vi "Unit Test.vi"() -> ()   [LabVIEW 2019, in "Fluidic Process.lvlib"]
uses:
  Fluidic Process.lvlib
  SubVI/Fluidic Para.ctl
  User Event/Controls/UE Abort Action.ctl
  <vilib>/Utility/file.llb/Read Delimited Spreadsheet (string).vi
  Syringe Pump/NE-500/NE-500.lvlib
  Selection Valve/IDEX/IDEX.lvlib
  LED/LED.lvlib
  IO/sbRIO9623/sbRIO9623.lvlib
panel:
  out "Force Sensor":bool
  out "Air Sealing":bool
  out "Total Process":string
  out "Current Process":string
  out "Remaining Time(s)":dbl
  out "Gauge":dbl(knob)=1.2869315802184793e-48 scale=0.0..101.0
  in  "File Path":path
  in  "Fluidic Para":T1
  in  "Stop":bool
  in  "Run":bool
  out "Syringe Pump":bool
  out "Selection Valve":bool
  out "LED":bool
  out "I/O":bool
  in  "Open":bool
  # "/"
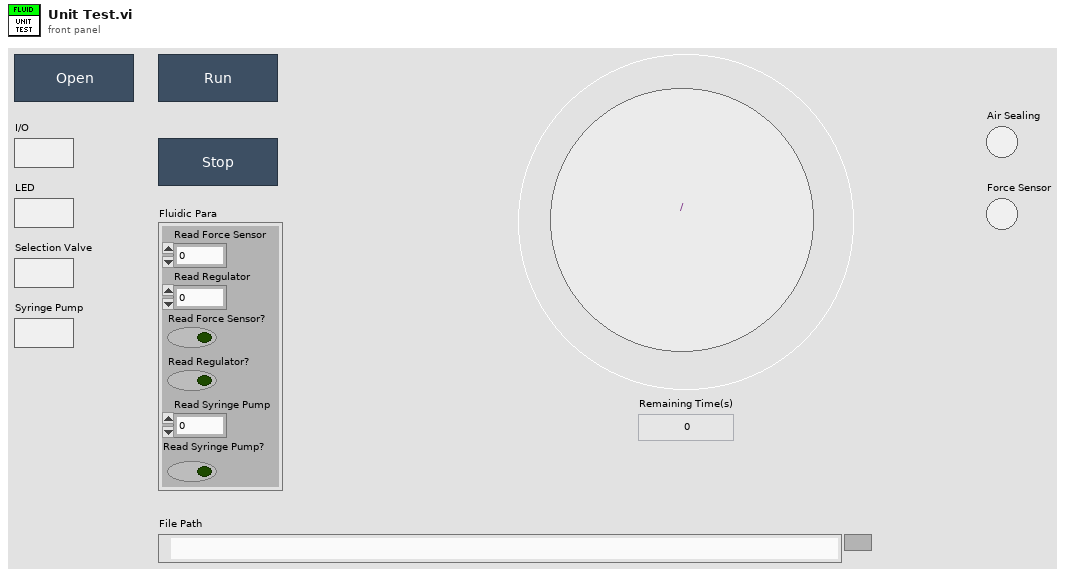
[diagram p1: front panel]
types:
  T1 = typedef "Fluidic Process.lvlib/Fluidic Para.ctl" = cluster{"Read Force Sensor":i32, "Read Regulator":i32, "Read Force Sensor?":bool, "Read Regulator?":bool, "Read Syringe Pump":i32, "Read Syringe Pump?":bool}
  T2 = typedef "UE Abort Action.ctl" = enum16{"Create", "Get", "Destroy"}
  T3 = typedef "Fluidic Process.lvlib/SEQ Data.ctl" = cluster{"Fluidic Process Done?":bool, "Current Process":i32, "Remaining Time":dbl, "Total Process":i32, "Air Sealing":bool, "Force Condition":bool}
  T4 = typedef "sbRIO9623.lvlib/SEQ Data.ctl" = cluster{"Lid Sensor 1":bool, "Lid Sensor 2":bool, "Laser Interlock":bool, "Buffer Tank":bool, "Wash Tank":bool, "Waste Tank":bool, "SiPM 1":fxp<+,20,5>, "SiPM 2":fxp<+,20,5>, "Initialize Success?":bool, "VI Refnum":refnum<vi>}
  T5 = typedef "LED.lvlib/SEQ Data.ctl" = cluster{"Initialize Sucess?":bool, "BL2 Regulator":dbl, "BL1 Regulator":dbl, "Blood Sensor 1":dbl, "Blood Sensor 2":dbl, "Air Pressure Sensor":dbl, "Force Snesor 1":u32, "Force Snesor 2":u32, "VI Refnum":refnum<vi>}
  T6 = typedef "IDEX.lvlib/SEQ Data.ctl" = cluster{"Position":string, "Initialize Done?":bool, "VI Refnum":refnum<vi>}
  T7 = typedef "NE-500.lvlib/SEQ Data.ctl" = cluster{"Status":string, "Initialize Done?":bool, "VI Refnum":refnum<vi>}
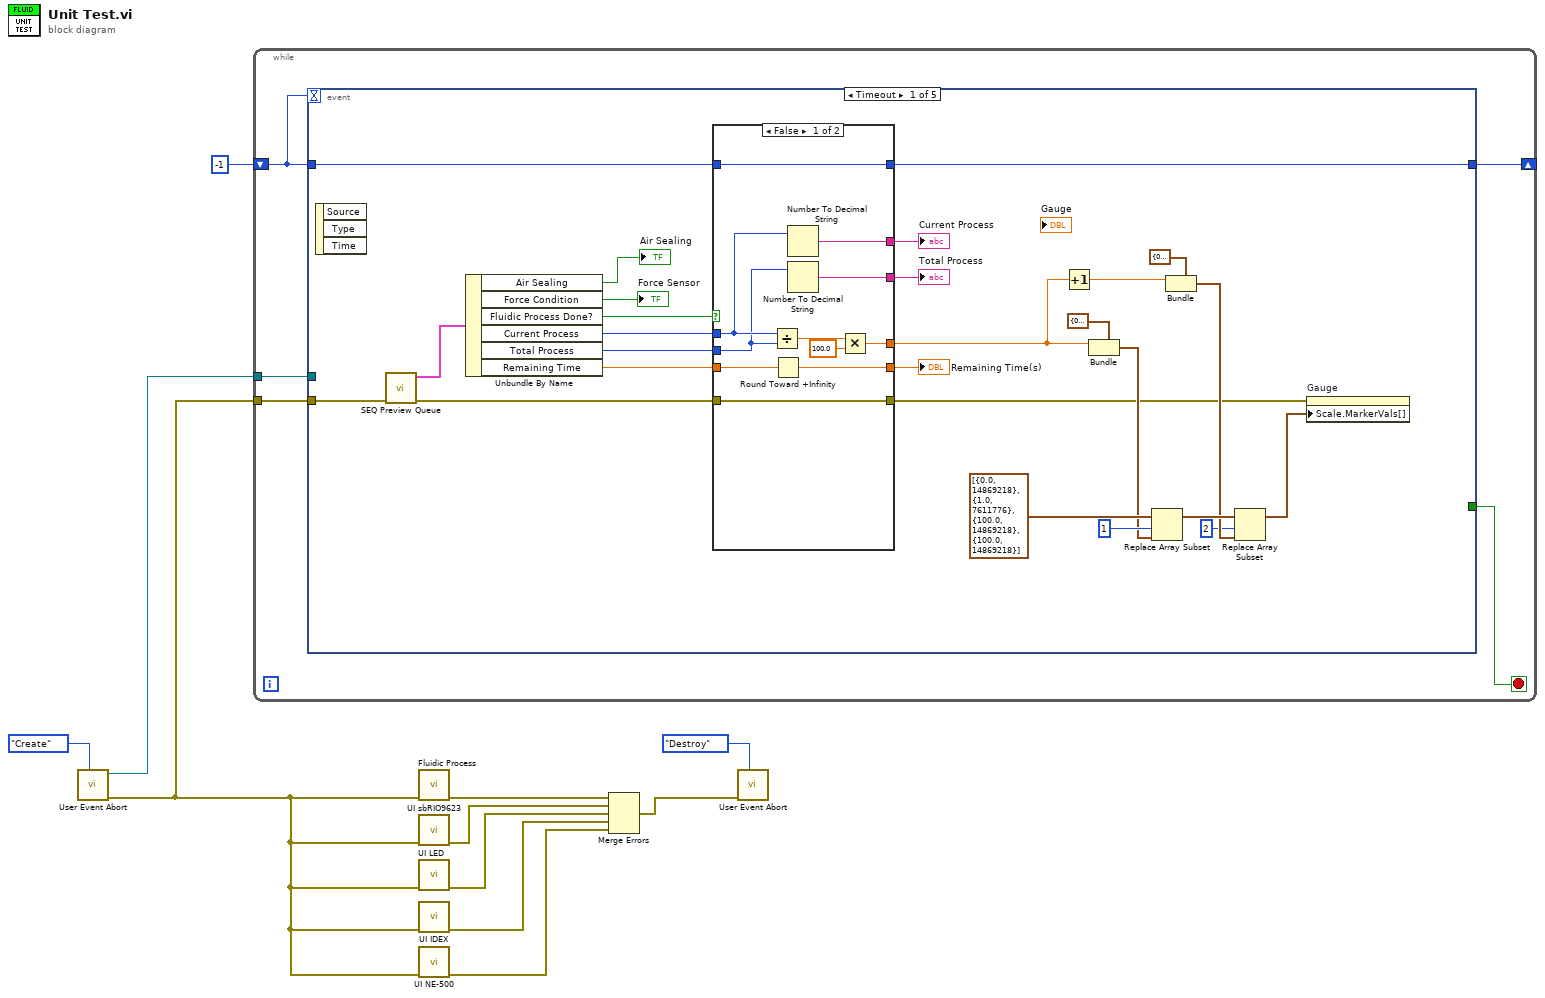
[diagram p0: block diagram]
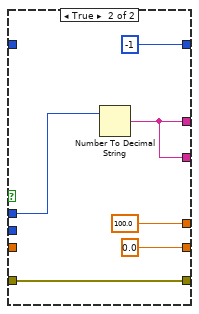
[diagram p2: hidden frame]
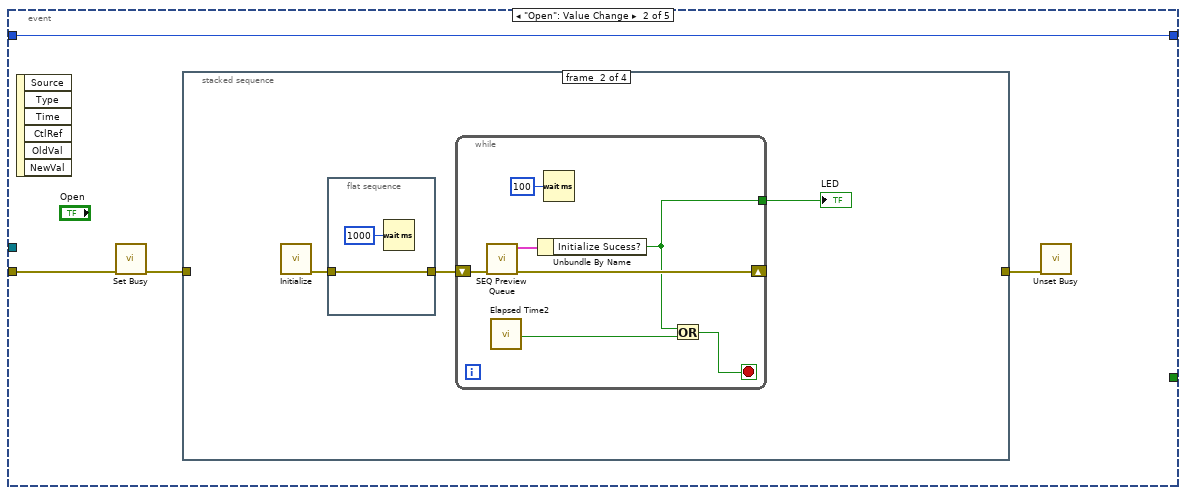
[diagram p3: hidden frame]
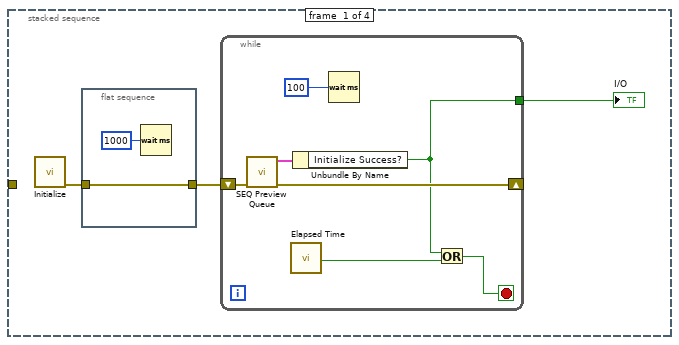
[diagram p4: hidden frame]
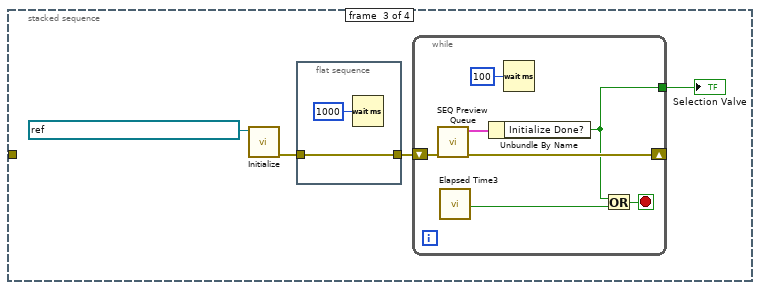
[diagram p5: hidden frame]
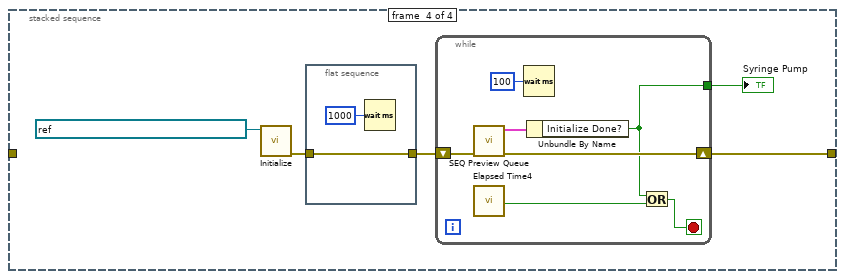
[diagram p6: hidden frame]
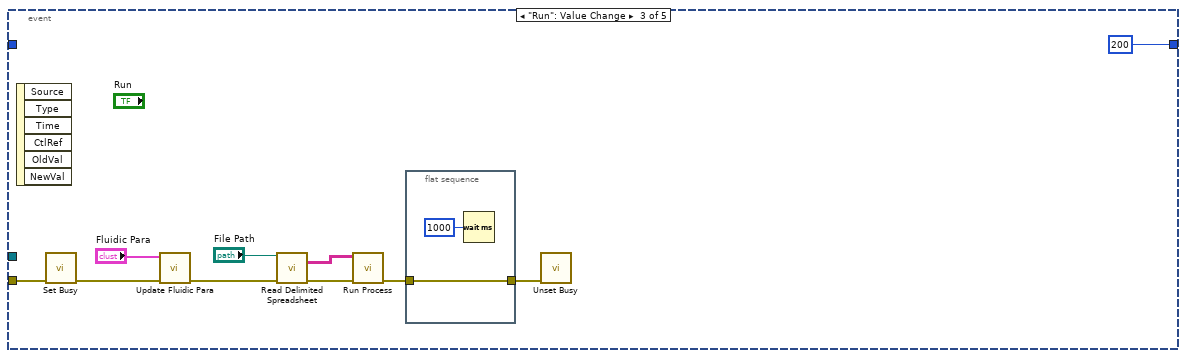
[diagram p7: hidden frame]
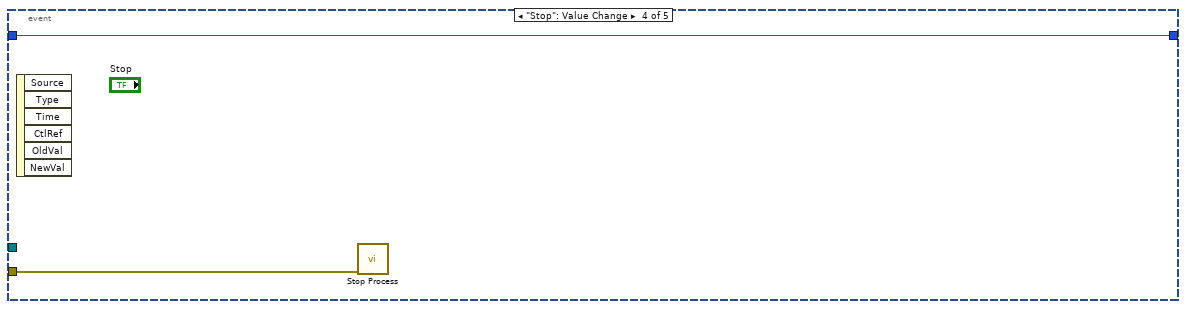
[diagram p8: hidden frame]
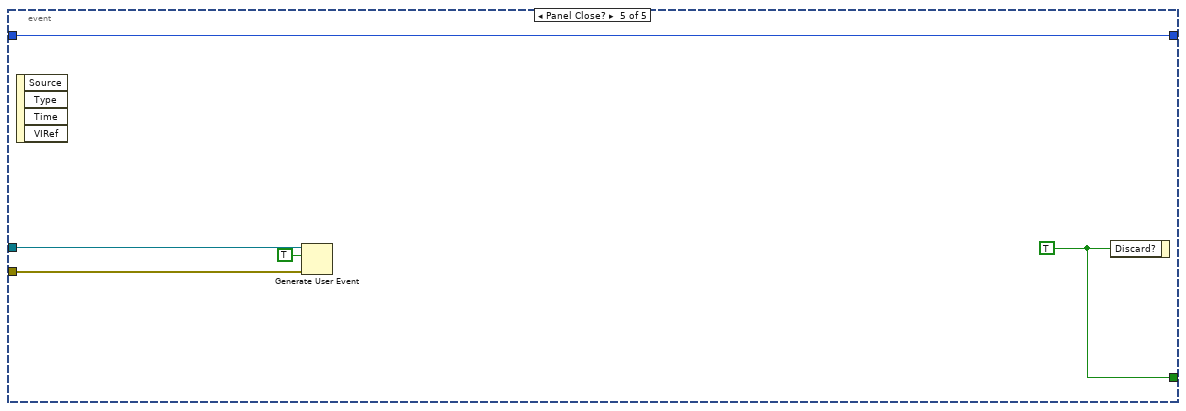
[diagram p9: hidden frame]
diagram:
  n1 = call "User Event Abort.vi"("Action"=UE_Abort_Action."Create") -> ("Error Out"=w2:errorcluster, "User Event Out"=w3:refnum<user-event>)  [unwired: 9 in]
  n2 = while {
    tunnel: w3 -> [w16]
    tunnel: w2 -> [w15]
    shift-right: [w13] -> _
    shift-left: -1 -> [w12]
    stop <- w14 stop-if-true
    n3 = event shown="[0] Timeout" {
      selector: _ -> [_ _ _ _ _]
      dyn-events: _ -> [_ _ _ _ _]
      timeout: w12 -> [_ _ _ _ _]
      tunnel: w16 -> [_ _ _ _ w133]
      tunnel: w15 -> [w42 w63 w118 w127 w132]
      tunnel: [_ _ _ _ w130] -> w14
      tunnel: w12 -> [w35 w60 _ w128 w129]
      tunnel: [w34 w60 200 w128 w129] -> w13
      event Timeout {
        n4 = event-data() -> ()  [unwired: 1 in, 3 out]
        n5 = call "SEQ Preview Queue.vi"("error in"=w42) -> ("error out"=w40:errorcluster, "SEQ Data"=w41:T3)  [unwired: 9 in]
        n6 = Unbundle By Name(w41) -> ("Air Sealing"=→"Air Sealing":bool, "Force Condition"=→"Force Sensor":bool, "Fluidic Process Done?"=w39:bool, "Current Process"=w38:i32, "Total Process"=w37:i32, "Remaining Time"=w36:dbl)
        n7 = case shown="False" w39 {
          tunnel: w40 -> [w49 w56]
          tunnel: w38 -> [w48 w55]
          tunnel: w37 -> [w46 _]
          tunnel: w36 -> [w44 _]
          tunnel: [w43 0.0 ("Remaining Time")] -> w21
          tunnel: [w51 100.0] -> w23
          tunnel: w35 -> [w50 _]
          tunnel: [w50 -1] -> w34
          tunnel: [w49 w56] -> w22
          tunnel: [w47 w54] -> w20
          tunnel: [w45 w54] -> w19
          frame False {
            n8 = Divide(x=w48, y=w46) -> (x/y=w53:dbl)
            n9 = Round Toward +Infinity(x=w44) -> (ceil(x): smallest int >= x=w43:dbl)
            n10 = Number To Decimal String(number=w48) -> (decimal integer string=w47:string)  [unwired: 1 in]
            n11 = Number To Decimal String(number=w46) -> (decimal integer string=w45:string)  [unwired: 1 in]
            n12 = Multiply(x=w53, y=100.0) -> (x*y=w51:dbl)
          }
          frame True {
            n13 = Number To Decimal String(number=w55) -> (decimal integer string=w54:string)  [unwired: 1 in]
          }
        }
        "Remaining Time(s)" <- w21
        "Current Process" <- w20
        "Total Process" <- w19
        n14 = Increment(x=w23) -> (x+1=w29:dbl)
        n15 = Bundle(cluster=cluster{dbl, i32} {0.0, 7611776}, w23) -> (w31:cluster{dbl, i32})  [unwired: 1 in]
        n16 = Replace Array Subset(array=cluster{dbl, u32}[] [{0.0, 14869218}, {1.0, 7611776}, {100.0, 14869218}, {100.0, 14869218}] ("Scale.Marker Values[]"), new element=w31, index=1) -> (w27:cluster{dbl, u32}[])
        n17 = Bundle(cluster=cluster{dbl, i32} {0.0, 14869218}, w29) -> (w26:cluster{dbl, i32})  [unwired: 1 in]
        n18 = Replace Array Subset(array=w27, new element=w26, index=2) -> (w24:cluster{dbl, u32}[])
        n19 = property on="Gauge" class="Knob (strict)"(error in=w22, "Scale.MarkerVals[]"=w24) -> ()  [unwired: 1 in, 2 out]
      }
      event "Open": Value Change {
        n20 = event-data() -> ()  [unwired: 1 in, 6 out]
        n21 = call <vilib>:"Set Busy.vi"("error in (no error)"=w63) -> ("error out"=w62:errorcluster)  [unwired: 9 in, 1 out]
        n22 = stacked-sequence {
          tunnel: w62 -> [_ _ _ _]
          tunnel: [_ _ _ w103] -> w61
          frame #0 {
            n23 = call "Initialize.vi"() -> ("Error Out"=w66:errorcluster)  [unwired: 11 in]
            n24 = flat-sequence {
              tunnel: w66 -> [w74]
              tunnel: [w74] -> w65
              frame #0 {
                n25 = Wait (ms)(milliseconds to wait=u32 1000) -> ()  [unwired: 1 out]
              }
            }
            n26 = while {
              shift-right: [w72] -> _
              shift-left: w65 -> [w73]
              tunnel: [w68] -> w64
              stop <- w67 stop-if-true
              n27 = call "SEQ Preview Queue.vi"("error in"=w73) -> ("error out"=w72:errorcluster, "SEQ Data"=w71:T4)  [unwired: 9 in]
              n28 = call "Elapsed Time"() -> ("Time has Elapsed"=w70:bool)  [unwired: 12 in, 7 out]
              n29 = Unbundle By Name(w71) -> ("Initialize Success?"=w68:bool)
              n30 = Wait (ms)(milliseconds to wait=u32 100) -> ()  [unwired: 1 out]
              n31 = Or(x=w68, y=w70) -> (x .or. y?=w67:bool)
            }
            "I/O" <- w64
          }
          frame #1 {
            n32 = call "Initialize.vi"() -> ("Error Out"=w78:errorcluster)  [unwired: 11 in]
            n33 = flat-sequence {
              tunnel: w78 -> [w86]
              tunnel: [w86] -> w77
              frame #0 {
                n34 = Wait (ms)(milliseconds to wait=u32 1000) -> ()  [unwired: 1 out]
              }
            }
            n35 = while {
              shift-right: [w83] -> _
              shift-left: w77 -> [w85]
              tunnel: [w80] -> w76
              stop <- w79 stop-if-true
              n36 = call "SEQ Preview Queue.vi"("error in"=w85) -> ("error out"=w83:errorcluster, "SEQ Data"=w82:T5)  [unwired: 9 in]
              n37 = call "Elapsed Time2"() -> ("Time has Elapsed"=w81:bool)  [unwired: 12 in, 7 out]
              n38 = Unbundle By Name(w82) -> ("Initialize Sucess?"=w80:bool)
              n39 = Wait (ms)(milliseconds to wait=u32 100) -> ()  [unwired: 1 out]
              n40 = Or(x=w80, y=w81) -> (x .or. y?=w79:bool)
            }
            "LED" <- w76
          }
          frame #2 {
            n41 = call "Initialize.vi"("VISA name"=refnum<visa-resource-name> "visa://169.254.25.118/ASRL1::INSTR") -> ("Error Out"=w91:errorcluster)  [unwired: 10 in]
            n42 = flat-sequence {
              tunnel: w91 -> [w92]
              tunnel: [w92] -> w90
              frame #0 {
                n43 = Wait (ms)(milliseconds to wait=u32 1000) -> ()  [unwired: 1 out]
              }
            }
            n44 = while {
              tunnel: [w94] -> w89
              shift-right: [w97] -> _
              shift-left: w90 -> [w99]
              stop <- w95 stop-if-true
              n45 = call "SEQ Preview Queue.vi"("error in"=w99) -> ("error out"=w97:errorcluster, "SEQ Data"=w98:T6)  [unwired: 9 in]
              n46 = call "Elapsed Time3"() -> ("Time has Elapsed"=w96:bool)  [unwired: 12 in, 7 out]
              n47 = Unbundle By Name(w98) -> ("Initialize Done?"=w94:bool)
              n48 = Wait (ms)(milliseconds to wait=u32 100) -> ()  [unwired: 1 out]
              n49 = Or(x=w94, y=w96) -> (x .or. y?=w95:bool)
            }
            "Selection Valve" <- w89
          }
          frame #3 {
            n50 = call "Initialize.vi"("VISA name"=refnum<visa-resource-name> "visa://169.254.25.118/ASRL2::INSTR") -> ("Error Out"=w105:errorcluster)  [unwired: 10 in]
            n51 = flat-sequence {
              tunnel: w105 -> [w107]
              tunnel: [w107] -> w104
              frame #0 {
                n52 = Wait (ms)(milliseconds to wait=u32 1000) -> ()  [unwired: 1 out]
              }
            }
            n53 = while {
              shift-right: [w112] -> w103
              shift-left: w104 -> [w114]
              tunnel: [w108] -> w101
              stop <- w109 stop-if-true
              n54 = call "SEQ Preview Queue.vi"("error in"=w114) -> ("error out"=w112:errorcluster, "SEQ Data"=w113:T7)  [unwired: 9 in]
              n55 = call "Elapsed Time4"() -> ("Time has Elapsed"=w110:bool)  [unwired: 12 in, 7 out]
              n56 = Wait (ms)(milliseconds to wait=u32 100) -> ()  [unwired: 1 out]
              n57 = Unbundle By Name(w113) -> ("Initialize Done?"=w108:bool)
              n58 = Or(x=w108, y=w110) -> (x .or. y?=w109:bool)
            }
            "Syringe Pump" <- w101
          }
        }
        n59 = call <vilib>:"Unset Busy.vi"("error in (no error)"=w61) -> ()  [unwired: 10 in, 1 out]
      }
      event "Run": Value Change {
        n60 = event-data() -> ()  [unwired: 1 in, 6 out]
        n61 = call <vilib>:"Set Busy.vi"("error in (no error)"=w118) -> ("error out"=w117:errorcluster)  [unwired: 9 in, 1 out]
        n62 = call "Update Fluidic Para.vi"("Error In"=w117, "Fluidic Para"="Fluidic Para") -> ("Error Out"=w123:errorcluster)  [unwired: 9 in]
        n63 = call-poly <vilib>:"Read Delimited Spreadsheet.vi"("file path (dialog if empty)"="File Path", "error in (no error)"=w123) -> ("all rows"=w120:string[][], "error out"=w122:errorcluster)  [unwired: 8 in, 4 out]
        n64 = call "Run Process.vi"("Error In"=w122, "Fluidic Process in"=w120) -> ("Error Out"=w119:errorcluster)  [unwired: 9 in]
        n65 = flat-sequence {
          tunnel: w119 -> [w125]
          tunnel: [w125] -> w116
          frame #0 {
            n66 = Wait (ms)(milliseconds to wait=u32 1000) -> ()  [unwired: 1 out]
          }
        }
        n67 = call <vilib>:"Unset Busy.vi"("error in (no error)"=w116) -> ()  [unwired: 10 in, 1 out]
      }
      event "Stop": Value Change {
        n68 = event-data() -> ()  [unwired: 1 in, 6 out]
        n69 = call "Stop Process.vi"("Error In"=w127) -> ()  [unwired: 10 in, 1 out]
      }
      event Panel Close? {
        w130 = TRUE
        n70 = event-data() -> ()  [unwired: 1 in, 4 out]
        n71 = Generate User Event(user event=w133, event data cluster=TRUE ("event data"), error in=w132) -> ()  [unwired: 1 in, 2 out]
        n72 = event-data("Discard?"=w130) -> ()  [unwired: 1 in, 1 out]
      }
    }
  }
  n73 = call "Fluidic Process.vi"("error in"=w2) -> ("error out"=w9:errorcluster)  [unwired: 10 in]
  n74 = call "UI sbRIO9623.vi"("error in"=w2) -> ("error out"=w7:errorcluster)  [unwired: 10 in]
  n75 = call "UI LED.vi"("error in"=w2) -> ("error out"=w6:errorcluster)  [unwired: 10 in]
  n76 = call "UI IDEX.vi"("error in"=w2) -> ("error out"=w5:errorcluster)  [unwired: 10 in]
  n77 = call "UI NE-500.vi"("error in"=w2) -> ("error out"=w4:errorcluster)  [unwired: 10 in]
  n78 = Merge Errors(w9, w7, w6, w5, w4) -> (w8:errorcluster)
  n79 = call "User Event Abort.vi"("Action"=UE_Abort_Action."Destroy", "Error In"=w8) -> ()  [unwired: 8 in, 2 out]
